vi "AudioStreamer.EnumerateMicrophones.vi"() -> (0 "devices":string[](array[string]))   [LabVIEW 2020]
uses:
  <vilib>/Dataflow_G/G-Audio/G-Audio.lvlib
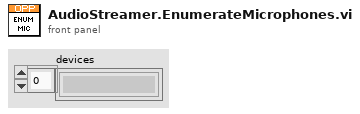
[diagram p1: front panel]
types:
  T1 = typedef "G-Audio.lvlib/Audio Device Info.ctl" = cluster{"Name":string, "ID":u8[], "Device Type":T2, "Default":bool, "Native Data Formats":T3[]}
  T2 = typedef "G-Audio.lvlib/Audio Device Type.ctl" = enum16{"(None)", "Playback", "Capture", "Duplex", "Loopback"}
  T3 = typedef "G-Audio.lvlib/Audio Device Native Data Format.ctl" = cluster{"Format":T4, "Channels":u32, "Sample Rate (Hz)":u32, "Exclusive Mode":bool}
  T4 = typedef "G-Audio.lvlib/Audio Device Format.ctl" = enum16{"Native", "U8", "I16", "I32", "SGL"}
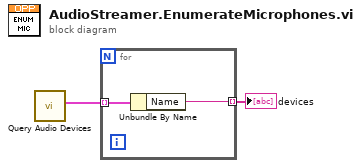
[diagram p0: block diagram]
diagram:
  n1 = call <vilib>:"Query Audio Devices.vi"() -> ("Capture Devices"=w2:T1[])  [unwired: 7 in, 4 out]
  n2 = for {
    tunnel: w2 -> [w4] mode=indexing
    tunnel: [w3] -> w1 mode=indexing
    n3 = Unbundle By Name(w4) -> ("Name"=w3:string)
  }
  "devices" <- w1
